vi "CRYCalc Impedance Mic Current.vi"(4 "Signal Type Input Name":string, 6 "Auto Mode":u16, 8 "Mic Ref resistor":dbl, 9 "Impedance":bool, 10 "Resistor value(Rref)":dbl format="%.2f", 11 "Freq resp curves(Vref)":cluster{cluster{"x":dbl, "y":dbl, "z":dbl}[]}[](array[cluster]) {"?"."z" format="%.2f"; "?"."y" format="%.2f"; "?"."x" format="%.2f"}) -> (3 "Freq resp curves out":cluster{cluster{"x":dbl, "y":dbl, "z":dbl}[]}[](array[cluster]) {"?"."z" format="%.2f"; "?"."y" format="%.2f"; "?"."x" format="%.2f"})   [LabVIEW 2013]
uses:
  <vilib>/Analysis/baseanly.llb/Mean (DBL).vi
  Hardware/CRYHardware Global.vi
  CRYProject/CRYProject Editor Global.vi
  <vilib>/Analysis/NI_AALBase.lvlib
panel:
  out "XY Graph":cluster{dbl[], dbl[]}(graph)
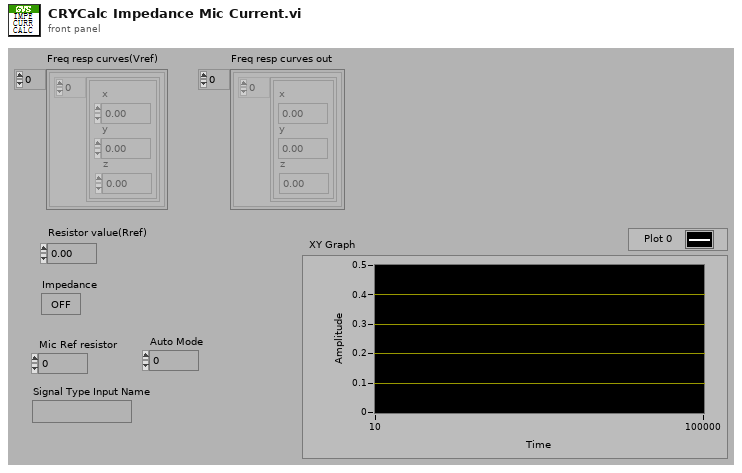
[diagram p1: front panel]
types:
  T1 = typedef "CRYStep.ctl" = cluster{"No.VI":i32, "Category":string, "StepName":string, "Seq setup flattened":string, "Comment":string, "Steps config.":bool[], "Jump config":i32[], "Start":dbl, "Increment":dbl, "Name":string, "Unit":string, "Y data":u16, "Y prefix":string, "Y dB ref":dbl, "Y unit":string, "Repeat State Array":cluster{"Start":dbl, "Increment":dbl, "Count":i32, "Num":i32}[]}
  T2 = typedef "CRYCalibration All Cluster.ctl" = cluster{"Calibration 2D":T3[], "Help":string, "Tab Value":i32, "Input Signal Type":string, "Output Signal Type":string}
  T3 = typedef "CRYCalibration 2DCluster.ctl" = cluster{"Calibration":T4, "Corr Curve":T5, "EQ Curve":T5, "Sens Curve":T5}
  T4 = typedef "CRYCalibration Cluster.ctl" = cluster{"Calibration Step Name":string, "Device":string, "Correction Curve Name":string, "Equalization Curve Name":string, "Sensitivity Curve Name":string, "Corr Folder and File":string, "EQ Folder and File":string, "Sens Folder and File":string, "Corr Step size":u16, "EQ Step size":u16, "Input":bool, "Last Cal Date (sec)":timestamp, "Cha Name":string, "Corr Curve Found":bool, "EQ Curve Found":bool, "Sens Curve Found":bool, "Signal Type":string, "Calibrated Device":string, "Hz":u32}
  T5 = typedef "CRYData Cluster.ctl" = cluster{"Name":string, "Curve":cluster{"x":dbl, "y":dbl, "z":dbl}[], "X data":u16, "Y data":u16, "Z data":u16, "X axis":u16, "Y axis":u16, "Z axis":u16, "X unit":string, "Y unit":string, "Z unit":string, "X dB ref":dbl, "Y dB ref":dbl, "Z dB ref":dbl, "single val":bool, "protected":bool, "display X":bool, "display Y":bool, "display Z":bool, "Test Info":string, "Step No.":i32, "Plot Settings":cluster{"Color":u32, "Interpolation":u8, "Point Style":u8, "Line Style":u8, "Point Color":u32, "Line Width":u8, "Bar Plot Style":u8, "Fill To":i16}, "AutoProtect":bool}
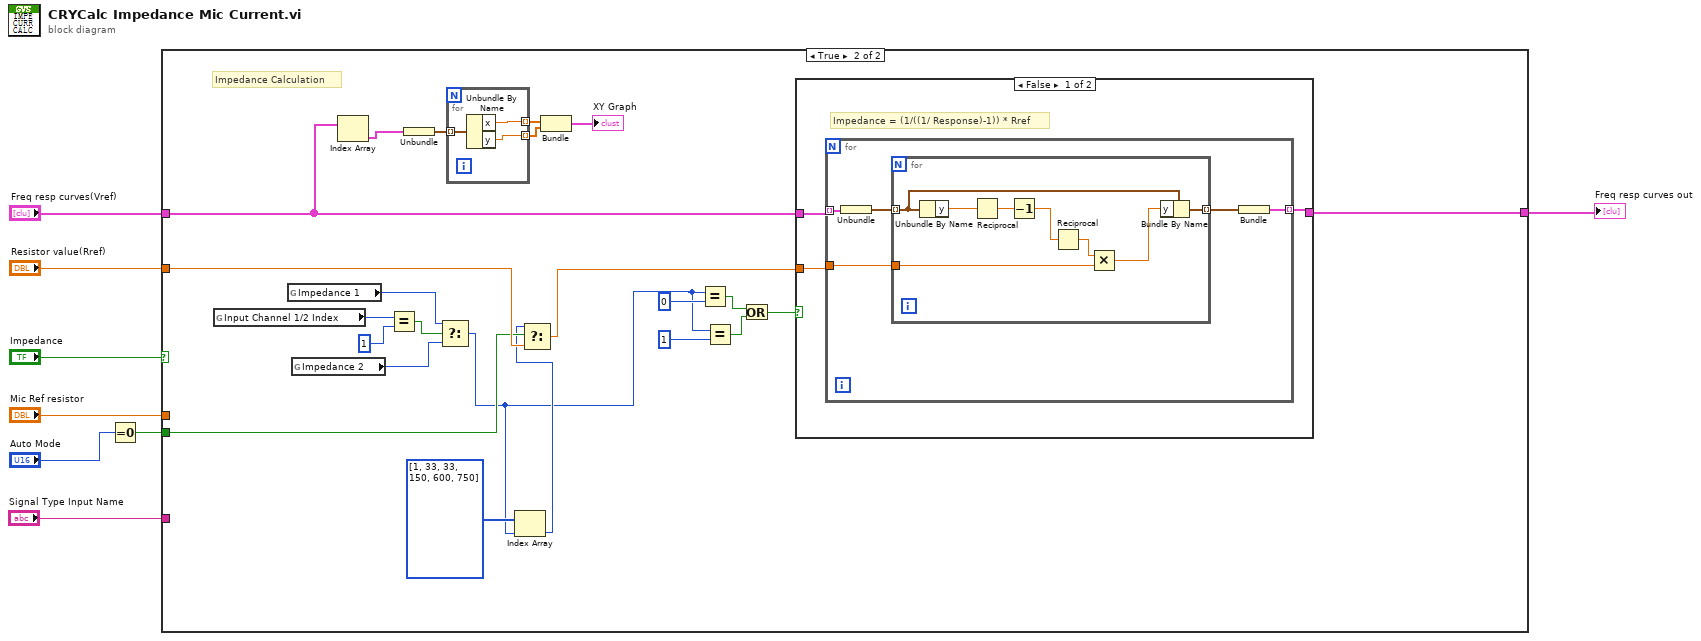
[diagram p0: block diagram]
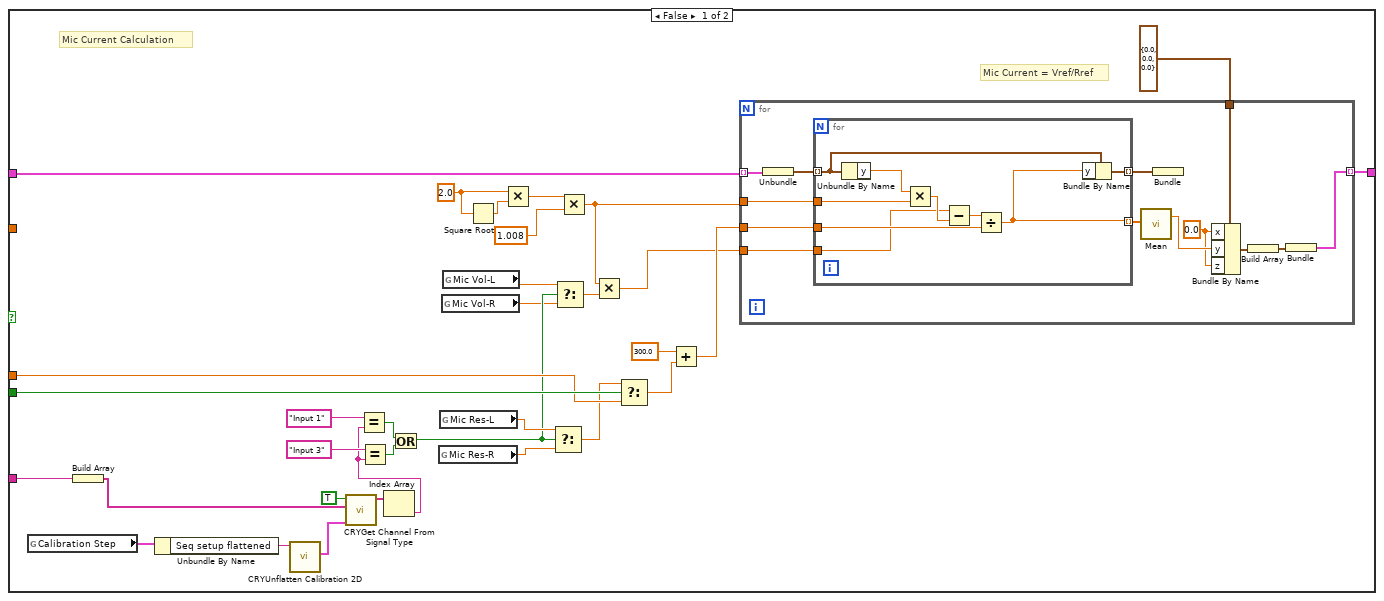
[diagram p2: hidden frame]
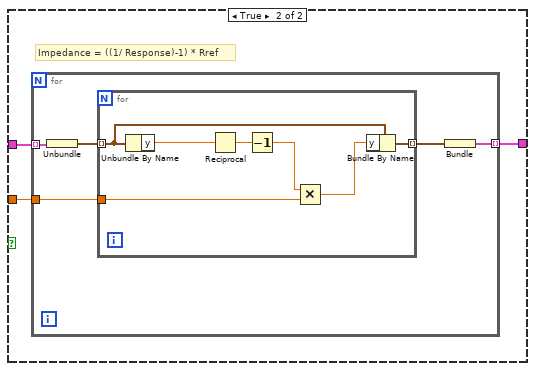
[diagram p3: hidden frame]
diagram:
  n1 = Equal To 0?(x="Auto Mode") -> (x = 0?=w3:bool)
  n2 = case shown="True" "Impedance" {
    tunnel: "Resistor value(Rref)" -> [_ w80]
    tunnel: [w40 w86] -> w7
    tunnel: "Freq resp curves(Vref)" -> [w41 w69]
    tunnel: w3 -> [w39 w78]
    tunnel: "Mic Ref resistor" -> [w38 _]
    tunnel: "Signal Type Input Name" -> [w28 _]
    frame False {
      w37 = 2.0 ("s? t:f")
      # "Mic Current Calculation"
      # "Mic Current = Vref/Rref"
      n3 = global read "CRYProject Editor Global.vi" "Calibration Step"() -> (w25:T1)
      n4 = Build Array(w28) -> (w27:string[])
      n5 = Unbundle By Name(w25) -> ("Seq setup flattened"=w24:string)
      n6 = call "CRYUnflatten Calibration 2D.vi"("Flattened Calibration"=w24) -> ("Calibration Step Out"=w23:T2)  [unwired: 8 in, 2 out]
      n7 = call "CRYGet Channel From Signal Type.vi"("Calibration"=w23, "Signal Type Name Array In"=w27, "In/Out?"=TRUE) -> ("Channel Name Array Out"=w22:string[])  [unwired: 7 in, 1 out]
      n8 = Index Array(array=w22) -> (element=w21:string)  [unwired: 1 in]
      n9 = Equal?(x="Input 1", y=w21) -> (x = y?=w31:bool)
      n10 = Equal?(x="Input 3", y=w21) -> (x = y?=w30:bool)
      n11 = Or(x=w31, y=w30) -> (x .or. y?=w17:bool)
      n12 = global read "CRYHardware Global.vi" "Mic Res-R"() -> (w33:dbl)
      n13 = global read "CRYHardware Global.vi" "Mic Res-L"() -> (w34:dbl)
      n14 = global read "CRYHardware Global.vi" "Mic Vol-R"() -> (w15:dbl)
      n15 = global read "CRYHardware Global.vi" "Mic Vol-L"() -> (w16:dbl)
      n16 = Square Root(x=w37) -> (sqrt(x)=w36:dbl)
      n17 = Multiply(x=w37, y=w36) -> (x*y=w13:dbl)
      n18 = Select(t=w34, s=w17, f=w33) -> (s? t:f=w29:dbl)
      n19 = Select(t=w16, s=w17, f=w15) -> (s? t:f=w12:dbl)
      n20 = Multiply(x=w13, y=1.008 ("x")) -> (x*y=w10:dbl)
      n21 = Multiply(x=w10, y=w12) -> (x*y=w11:dbl)
      n22 = Select(t=w29, s=w39, f=w38) -> (s? t:f=w20:dbl)
      n23 = Add(x=300.0, y=w20) -> (x+y=w18:dbl)
      n24 = for {
        tunnel: w41 -> [w54] mode=indexing
        tunnel: w18 -> [w52]
        tunnel: [w42] -> w40 mode=indexing
        tunnel: w10 -> [w50]
        tunnel: w11 -> [w49]
        tunnel: cluster{"x":dbl, "y":dbl, "z":dbl} {"x"=0.0, "y"=0.0, "z"=0.0} -> [w47]
        w45 = 0.0 ("x")
        n25 = Unbundle(w54) -> (w53:cluster{"x":dbl, "y":dbl, "z":dbl}[])
        n26 = for {
          tunnel: w53 -> [w63] mode=indexing
          tunnel: w52 -> [w61]
          tunnel: [w62] -> w51 mode=indexing
          tunnel: w50 -> [w59]
          tunnel: w49 -> [w57]
          tunnel: [w55] -> w48 mode=indexing
          n27 = Unbundle By Name(w63) -> ("y"=w60:dbl)
          n28 = Multiply(x=w60, y=w59) -> (x*y=w58:dbl)
          n29 = Subtract(x=w57, y=w58) -> (x-y=w56:dbl)
          n30 = Divide(x=w56, y=w61) -> (x/y=w55:dbl)
          n31 = Bundle By Name(cluster=w63, "y"=w55) -> (w62:cluster{"x":dbl, "y":dbl, "z":dbl})
        }
        n32 = call-poly <vilib>:"Mean.vi"("X"=w48) -> ("mean"=w46:dbl)  [unwired: 1 out]
        n33 = Bundle(w51) -> ()  [unwired: 1 in, 1 out]
        n34 = Bundle By Name(cluster=w47, "x"=w45, "y"=w46, "z"=w45) -> (w44:cluster{"x":dbl, "y":dbl, "z":dbl})
        n35 = Build Array(w44) -> (w43:cluster{"x":dbl, "y":dbl, "z":dbl}[])
        n36 = Bundle(w43) -> (w42:cluster{cluster{"x":dbl, "y":dbl, "z":dbl}[]})  [unwired: 1 in]
      }
    }
    frame True {
      # "Impedance Calculation"
      n37 = global read "CRYHardware Global.vi" "Input Channel 1/2 Index"() -> (w75:i32)
      n38 = global read "CRYHardware Global.vi" "Impedance 1"() -> (w72:i32)
      n39 = global read "CRYHardware Global.vi" "Impedance 2"() -> (w71:i32)
      n40 = Index Array(array=w69) -> (element=w68:cluster{cluster{"x":dbl, "y":dbl, "z":dbl}[]})  [unwired: 1 in]
      n41 = Equal?(x=w75, y=1) -> (x = y?=w73:bool)
      n42 = Unbundle(w68) -> (w67:cluster{"x":dbl, "y":dbl, "z":dbl}[])
      n43 = Select(t=w72, s=w73, f=w71) -> (s? t:f=w70:i32)
      n44 = for {
        tunnel: w67 -> [w89] mode=indexing
        tunnel: [w88] -> w66 mode=indexing
        tunnel: [w87] -> w65 mode=indexing
        n45 = Unbundle By Name(w89) -> ("x"=w88:dbl, "y"=w87:dbl)
      }
      n46 = Index Array(array=i32[] [1, 33, 33, 150, 600, 750], index=w70) -> (element=w76:i32)
      n47 = Select(t=w76, s=w78, f=w80) -> (s? t:f=w79:dbl)
      n48 = Bundle(w66, w65) -> (→"XY Graph":cluster{dbl[], dbl[]})  [unwired: 1 in]
      n49 = Equal?(x=w70, y=0 ("Impedance 1")) -> (x = y?=w83:bool)
      n50 = Equal?(x=w70, y=1 ("Impedance 1")) -> (x = y?=w82:bool)
      n51 = Or(x=w83, y=w82) -> (x .or. y?=w81:bool)
      n52 = case shown="False" w81 {
        tunnel: w79 -> [w91 w108]
        tunnel: [w90 w107] -> w86
        tunnel: w69 -> [w92 w106]
        frame False {
          # "Impedance = (1/((1/ Response)-1)) * Rref"
          n53 = for {
            tunnel: w92 -> [w97] mode=indexing
            tunnel: w91 -> [w95]
            tunnel: [w93] -> w90 mode=indexing
            n54 = Unbundle(w97) -> (w96:cluster{"x":dbl, "y":dbl, "z":dbl}[])
            n55 = for {
              tunnel: w96 -> [w105] mode=indexing
              tunnel: w95 -> [w101]
              tunnel: [w104] -> w94 mode=indexing
              n56 = Unbundle By Name(w105) -> ("y"=w103:dbl)
              n57 = Reciprocal(x=w103) -> (1/x=w102:dbl)
              n58 = Decrement(x=w102) -> (x-1=w99:dbl)
              n59 = Reciprocal(x=w99) -> (1/x=w98:dbl)
              n60 = Multiply(x=w98, y=w101) -> (x*y=w100:dbl)
              n61 = Bundle By Name(cluster=w105, "y"=w100) -> (w104:cluster{"x":dbl, "y":dbl, "z":dbl})
            }
            n62 = Bundle(w94) -> (w93:cluster{cluster{"x":dbl, "y":dbl, "z":dbl}[]})  [unwired: 1 in]
          }
        }
        frame True {
          # "Impedance = ((1/ Response)-1) * Rref"
          n63 = for {
            tunnel: w106 -> [w113] mode=indexing
            tunnel: w108 -> [w111]
            tunnel: [w109] -> w107 mode=indexing
            n64 = Unbundle(w113) -> (w112:cluster{"x":dbl, "y":dbl, "z":dbl}[])
            n65 = for {
              tunnel: w112 -> [w120] mode=indexing
              tunnel: w111 -> [w116]
              tunnel: [w119] -> w110 mode=indexing
              n66 = Unbundle By Name(w120) -> ("y"=w118:dbl)
              n67 = Reciprocal(x=w118) -> (1/x=w117:dbl)
              n68 = Decrement(x=w117) -> (x-1=w115:dbl)
              n69 = Multiply(x=w115, y=w116) -> (x*y=w114:dbl)
              n70 = Bundle By Name(cluster=w120, "y"=w114) -> (w119:cluster{"x":dbl, "y":dbl, "z":dbl})
            }
            n71 = Bundle(w110) -> (w109:cluster{cluster{"x":dbl, "y":dbl, "z":dbl}[]})  [unwired: 1 in]
          }
        }
      }
    }
  }
  "Freq resp curves out" <- w7
